vi "licdf record name.vi"(6 "out_record_size":i32, 7 "out_size":i32, 8 "error in (no error)":errorcluster, 9 "out":string, 10 "index":i32, 11 "handle":i32) -> (0 "error out":errorcluster, 1 "out out":string, 3 "function return":i32, 4 "out_record_size out":i32)   [LabVIEW 2026, in "keynub_licdongle.lvlib"]
doc: "int32_t licdf_record_name(int32_t handle, int32_t index, char *out, int32_t out_size,\n int32_t *out_record_size);"
uses:
  keynub_licdongle.lvlib
  natives/win-x64/keynub_licdongle_flat.dll
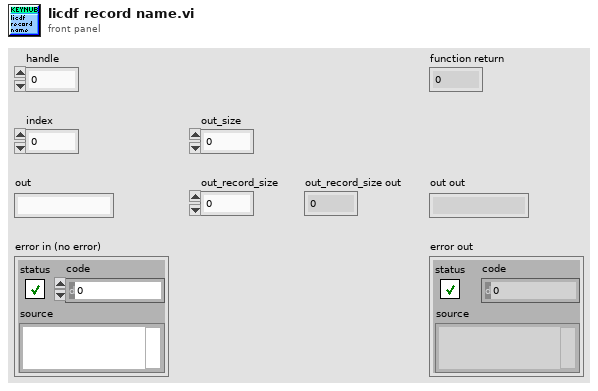
[diagram p1: front panel]
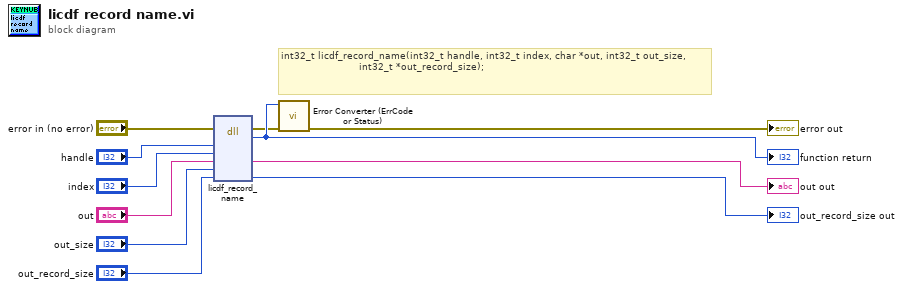
[diagram p0: block diagram]
diagram:
  # "int32_t licdf_record_name(int32_t handle, int32_t index, char *out, int32_t out_size,\n                          int32_t *out_record_size);"
  n1 = dll-call lib="C:/Austausch/KeyNub/LicenseDongle-PublicSDK/natives/win-x64/keynub_licdongle_flat.*" fn="licdf_record_name"(error in="error in (no error)", "handle"="handle", "index"="index", "out"="out", "out_size"="out_size", "out_record_size"="out_record_size") -> (error out=w2:errorcluster, w11:i32, "out"=→"out out":string, "out_record_size"=→"out_record_size out":i32)  [unwired: 5 in, 1 out]
  "function return" <- w11
  n2 = call "Error Converter (ErrCode or Status).vi"("error in (no error)"=w2, "error code"=w11) -> ("error out"=→"error out":errorcluster)  [unwired: 9 in]
